vi "Close.vi"(8 "error in":errorcluster, 11 "Acquire Continuous Waveform Configuration in":refnum<class "Continuous Waveform Acq CFG.lvclass">) -> (0 "error out":errorcluster, 3 "Acquire Continuous Waveform Configuration out":refnum<class "Continuous Waveform Acq CFG.lvclass">)   [LabVIEW 2023, in "RIGOL DS1054.lvlib" / "Continuous Waveform Acq CFG.lvclass"]
uses:
  Continuous Waveform Acq CFG.lvclass
  <instrlib>/RIGOL DS1000 Series/RIGOL DS1000 Series.lvlib
  Scope VISA/Configuration/Scope VISA CFG.lvclass
  D:/git/HAL/Scope VISA/Configuration/Scope VISA CFG.lvclass
  D:/git/HAL/Scope Base/Configuration/Scope Base CFG.lvclass
  D:/git/HAL/Configuration Base/Configuration Base.lvclass
  D:/git/HAL/Interfaces/IConfigure/IConfigure.lvclass
  D:/git/HAL/Devices/Rigol DS1054/Configurations/Acquire Continuous Waveform/Continuous Waveform Acq CFG.lvclass
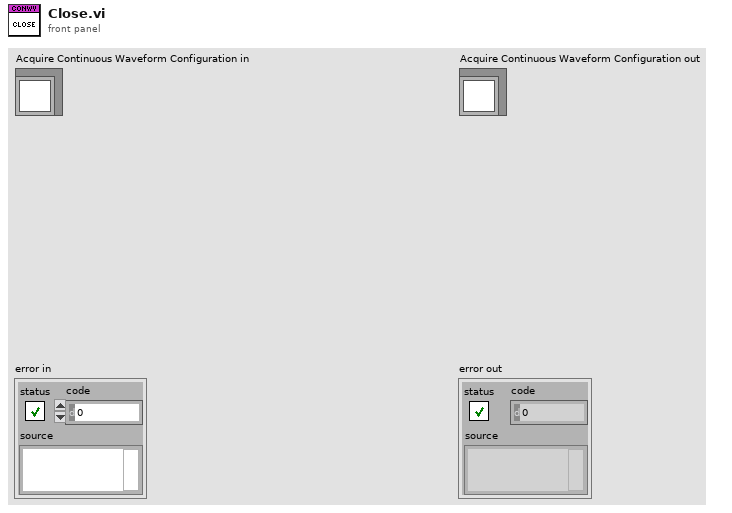
[diagram p1: front panel]
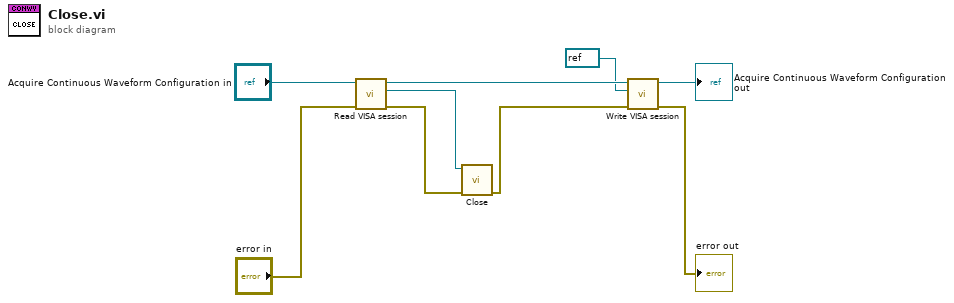
[diagram p0: block diagram]
diagram:
  n1 = call "Read VISA session.vi"("error in (no error)"="error in", "Scope VISA CFG in"="Acquire Continuous Waveform Configuration in") -> ("error out"=w7:errorcluster, "VISA session"=w5:refnum<visa-resource-name>, "Scope VISA CFG out"=w3:refnum<class "Continuous Waveform Acq CFG.lvclass">)  [unwired: 7 in]
  n2 = call <instrlib>:"Close.vi"("error in (no error)"=w7, "VISA resource name"=w5) -> ("error out"=w8:errorcluster)  [unwired: 9 out]
  n3 = call "Write VISA session.vi"("error in (no error)"=w8, "VISA session"=refnum<visa-resource-name> refnum, "Scope VISA CFG in"=w3) -> ("error out"=→"error out":errorcluster, "Scope VISA CFG out"=→"Acquire Continuous Waveform Configuration out":refnum<class "Continuous Waveform Acq CFG.lvclass">)  [unwired: 7 in]
